vi "HighFrameRateRecording.vi"() -> ()   [LabVIEW 2014]
doc: "The LL Ring VI acquires images continuously and displays them in an image control using the low-level acquisition VIs. A ring initiates a continuous high-speed acquisition to multiple buffers and is appropriate for high-speed applications that perform processing on every image. Multiple buffers are useful when processing times vary depending on other applications and processing results .\n\nIMAQ Init initializes the device. IMAQ Configure List configures the buffer list with multiple buffers. IMAQ Create creates the image buffers. Call IMAQ Configure Buffer once for each buffer in the buffer list. IMAQ Start starts the acquisition, and IMAQ Extract Buffer ensures that the current image is not overwritten. An image control displays the image on the front panel. After exiting the loop, IMAQ Extract Buffer releases the last extracted buffer. IMAQ Close releases resources associated with the acquisition, and IMAQ Dispose frees the image buffer."
uses:
  <vilib>/vision/Avi.llb/IMAQ AVI2 Refnum.ctl
  <vilib>/vision/Avi.llb/IMAQ AVI2 Codec Path.ctl
  SubVI/Global_Video_Frame_Number.vi
panel:
  in  "Frames per file":i32
  out "AVI Refnum":T1
  out "Video recording":bool
  in  "Record? (Home bt.)":bool
  in  "codec index":i32=5
  out "Error (%)":dbl format="%#.4g"
  out "Missing Frames":i32
  out "Frame Number":u32=17170882
  out "codec":string="Y800 Uncompressed Grey Scale (NI Vision)"
  in  "AVI File Path":path=path "E:/Video/test/30fps.avi"
  out "Processed Frames/s":dbl=30.00968054211036 format="%#.1g"
  in  "Stop":bool
  out "Saved Frames":i32
  out "Image":T2(plugin-control)
  in  "camera selection":string="img0"
  in  "Buffer size (frames)":u32=1000
  # "ToDo:\n - add JSON output\n - andd indicator of _s# number"
  # "1.  Initialisation"
  # "Codec should be:\n\"Y800 Uncompressed Grey Scale\""
  # "Naming convention:\n - use the name above and add _s#.avi for videos\n - specs for saved videos is specified in name.json"
  # "2.  Recording"
  # "y"
  # "Record"
  # "x"
  # "Just Observe"
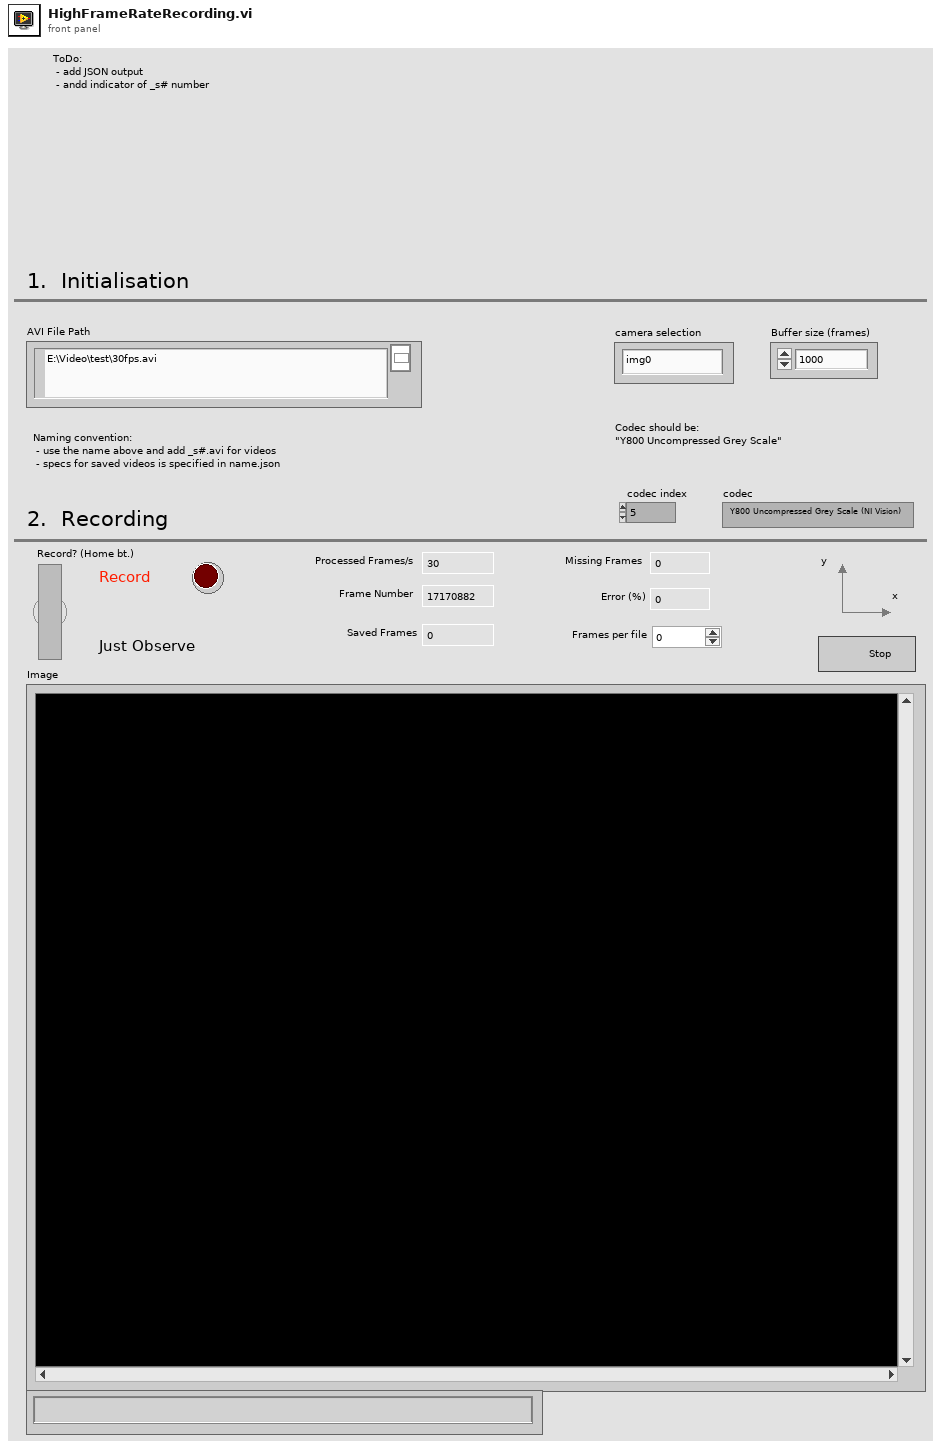
[diagram p1: front panel]
types:
  T1 = typedef "IMAQ AVI2 Refnum.ctl" = refnum<k20>
  T2 = typedef "IMAQ Image.ctl" = refnum<image>
  T3 = typedef "IMAQ AVI2 Codec Path.ctl" = u32
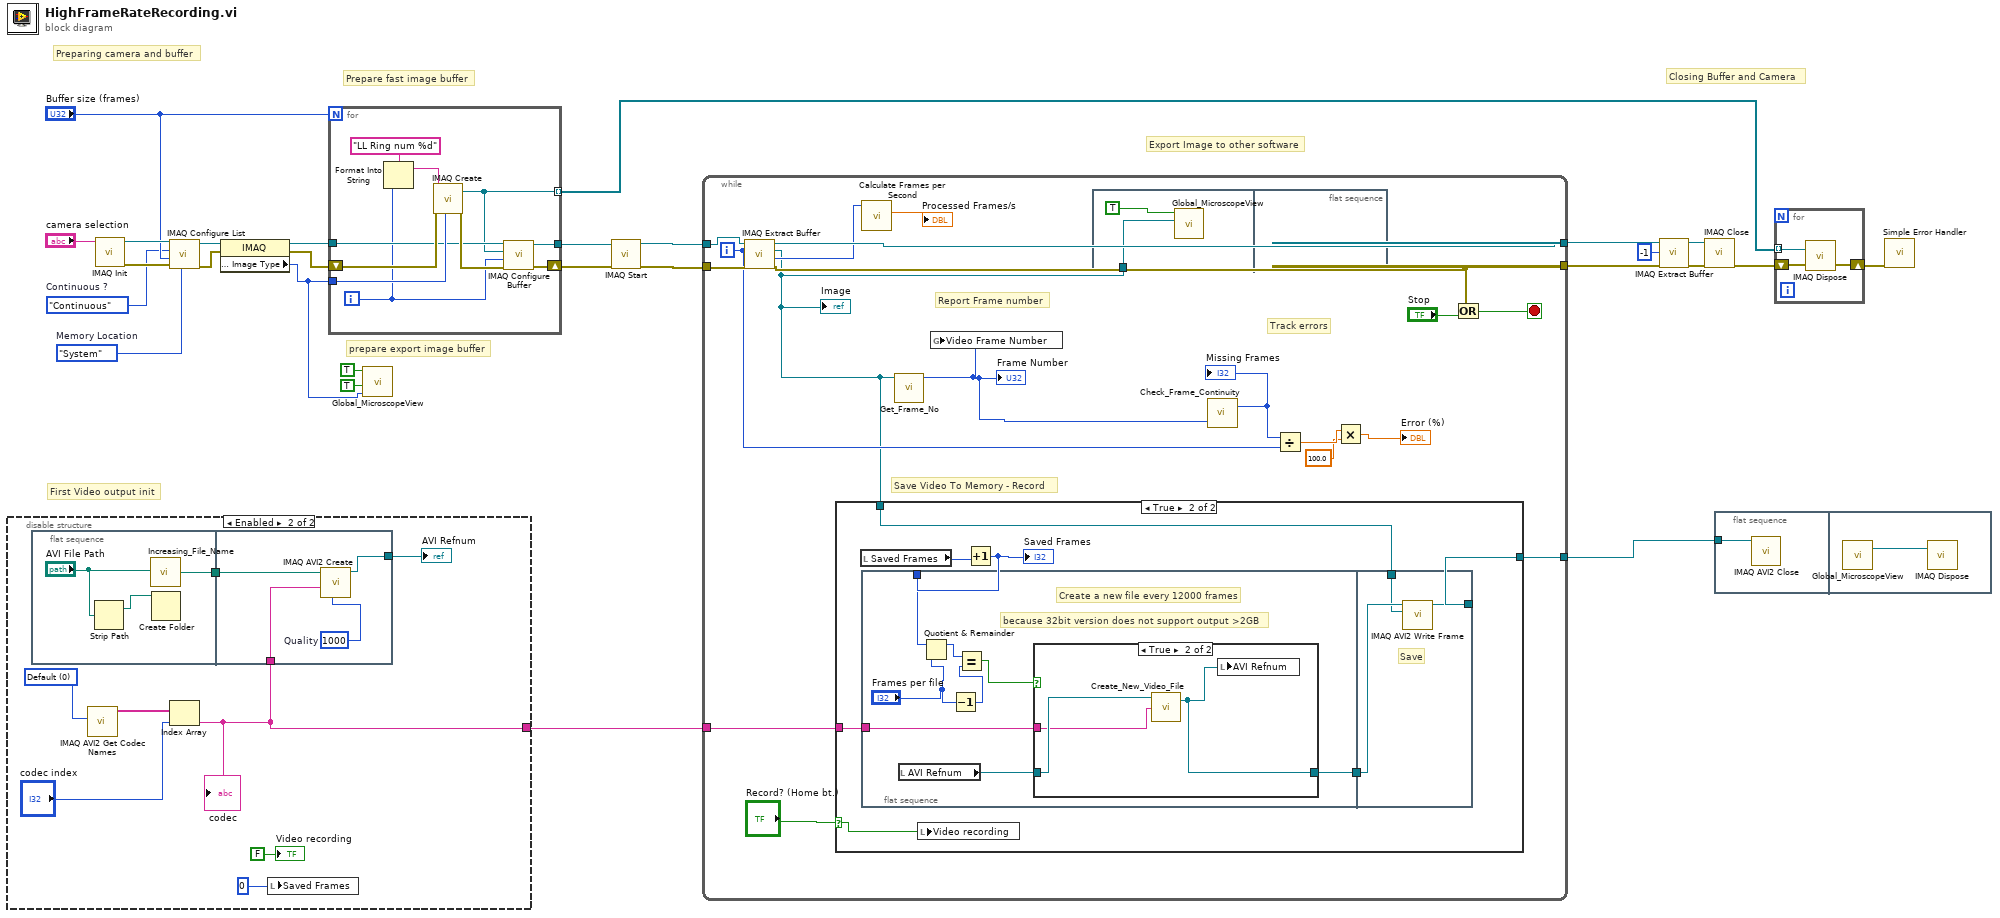
[diagram p0: block diagram]
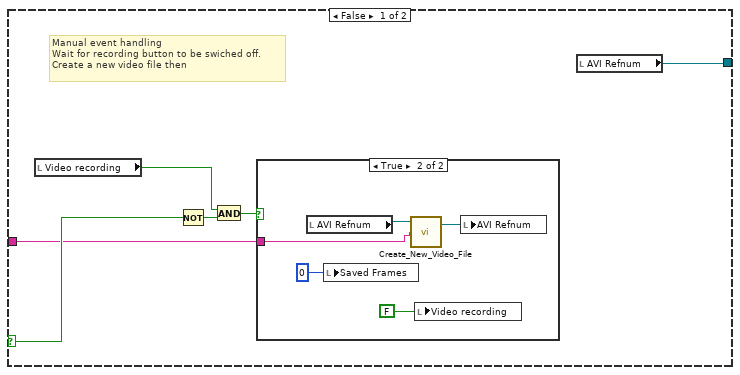
[diagram p3: hidden frame]
diagram:
  w9 = enum16{"System", "Onboard"}."System"  # Memory Location
  w8 = enum16{"One-Shot", "Continuous"}."Continuous"  # Continuous ?
  # "Export Image to other software"
  # "prepare export image buffer"
  # "Prepare fast image buffer"
  # "First Video output init"
  # "Closing Buffer and Camera"
  # "Preparing camera and buffer"
  n1 = disable-structure shown="Enabled" {
    disable-tunnel: [_ w28] -> w4
    frame Disabled {
    }
    frame Enabled {
      w35 = T3 0 items=["Default", "System", "Built in Vision"] ("Codec Source")
      n2 = flat-sequence {
        tunnel: [w38] -> w30
        tunnel: w30 -> [w40]
        tunnel: [w41] -> w29
        tunnel: w28 -> [w39]
        frame #0 {
          n3 = Strip Path(path="AVI File Path") -> (stripped path=w37:path)  [unwired: 1 out]
          n4 = call "Increasing_File_Name.vi"("Base AVI  path"="AVI File Path") -> ("Final AVI path"=w38:path)
          n5 = Create Folder(path (use dialog)=w37) -> ()  [unwired: 2 in, 3 out]
        }
        frame #1 {
          w42 = 1000  # Quality
          n6 = call "IMAQ AVI2 Create"("Quality"=w42, "Codec"=w39, "AVI Path"=w40) -> ("AVI Refnum"=w41:T1)  [unwired: 7 in, 1 out]
        }
      }
      n7 = call "IMAQ AVI2 Get Codec Names"("Codec Source"=w35) -> ("Codec Names"=w34:string[])  [unwired: 9 in, 1 out]
      n8 = Index Array(array=w34, index="codec index") -> (element=w28:string)
      "codec" <- w28
      n9 = local write "Saved Frames"(0 ("Saved Frames")) -> ()
      "AVI Refnum" <- w29
      "Video recording" <- FALSE ("Video recording")
    }
  }
  n10 = call <vilib>:"IMAQ Init.vi"("Interface Name"="camera selection") -> ("error out"=w26:errorcluster, "IMAQ Session Out"=w27:refnum<k11>)  [unwired: 1 in, 8 out]
  n11 = call <vilib>:"IMAQ Configure List.vi"("Memory Location"=w9, "error in (no error)"=w26, "Number of buffers"="Buffer size (frames)", "Continuous?"=w8, "IMAQ Session In"=w27) -> ("error out"=w22:errorcluster, "IMAQ Session Out"=w21:refnum<k11>)  [unwired: 1 in, 4 out]
  n12 = property class="IMAQ"(reference=w21, error in=w22) -> (reference out=w14:refnum<k11>, error out=w13:errorcluster, "Image Parameters : Image Type"=w1:u32)
  n13 = for {
    N: "Buffer size (frames)" -> [_]
    tunnel: [w52] -> w11
    tunnel: w1 -> [w50]
    tunnel: w14 -> [w47]
    shift-right: [w51] -> w10
    shift-left: w13 -> [w49]
    tunnel: [w43] -> w7 mode=indexing
    i -> [w44]
    n14 = Format Into String(format string="LL Ring num %d", w44) -> (resulting string=w46:string)  [unwired: 2 in, 1 out]
    n15 = call "IMAQ Create"("Image Name"=w46, "Image Type"=w50, "error in (no error)"=w49) -> ("New Image"=w43:T2, "error out"=w48:errorcluster)  [unwired: 1 in, 1 out]
    n16 = call <vilib>:"IMAQ Configure Buffer.vi"("error in (no error)"=w48, "Buffer Number"=w44, "Image In"=w43, "IMAQ Session In"=w47) -> ("error out"=w51:errorcluster, "IMAQ Session Out"=w52:refnum<k11>)  [unwired: 2 in, 4 out]
  }
  n17 = call "Global_MicroscopeView.vi"("Image Type"=w1, "Initialise"=TRUE, "Update Image"=TRUE) -> ()  [unwired: 1 in, 2 out]
  n18 = call <vilib>:"IMAQ Start.vi"("error in (no error)"=w10, "IMAQ Session In"=w11) -> ("error out"=w6:errorcluster, "IMAQ Session Out"=w17:refnum<k11>)  [unwired: 8 out]
  n19 = while {
    tunnel: [w68] -> w19
    tunnel: w17 -> [w69]
    tunnel: [w57] -> w18
    tunnel: w6 -> [w64]
    tunnel: [w56] -> w5
    tunnel: w4 -> [w55]
    i -> [w59]
    stop <- w70 stop-if-true
    # "Track errors"
    # "Report Frame number"
    # "Save Video To Memory - Record"
    n20 = call <vilib>:"IMAQ Extract Buffer.vi"("error in (no error)"=w64, "Buffer to extract"=w59, "IMAQ Session In"=w69) -> ("error out"=w57:errorcluster, "Buffer Number"=w65:i32, "Image Out"=w53:T2, "IMAQ Session Out"=w68:refnum<k11>)  [unwired: 5 out]
    "Image" <- w53
    n21 = case shown="True" "Record? (Home bt.)" {
      selector: "Record? (Home bt.)" -> [w75 w85]
      tunnel: [w78 w88] -> w56
      tunnel: w53 -> [_ w86]
      tunnel: w55 -> [w73 w84]
      frame False {
        # "Manual event handling\nWait for recording button to be swiched off.\nCreate a new video file then"
        n22 = local read "Video recording"() -> (w74:bool)
        n23 = Not(x=w75) -> (.not. x?=w76:bool)
        n24 = And(x=w74, y=w76) -> (x .and. y?=w77:bool)
        n25 = case shown="True" w77 {
          tunnel: w73 -> [_ w79]
          frame False {
          }
          frame True {
            n26 = local read "AVI Refnum"() -> (w82:T1)
            n27 = local write "Saved Frames"(0 ("Saved Frames")) -> ()
            n28 = call "Create_New_Video_File.vi"("Codec"=w79, "AVI Refnum IN"=w82) -> ("AVI Refnum OUT"=w83:T1)  [unwired: 1 in, 1 out]
            n29 = local write "Video recording"(FALSE ("Video recording")) -> ()
            n30 = local write "AVI Refnum"(w83) -> ()
          }
        }
        n31 = local read "AVI Refnum"() -> (w78:T1)
      }
      frame True {
        n32 = local read "Saved Frames"() -> (w90:i32)
        n33 = flat-sequence {
          tunnel: w89 -> [w96]
          tunnel: [w93] -> w87
          tunnel: w84 -> [w92]
          tunnel: [w105] -> w88
          tunnel: w87 -> [w104]
          tunnel: w86 -> [w103]
          frame #0 {
            # "because 32bit version does not support output >2GB"
            # "Create a new file every 12000 frames"
            n34 = local read "AVI Refnum"() -> (w94:T1)
            n35 = Quotient & Remainder(x=w96, y="Frames per file") -> (x-y*floor(x/y)=w98:i32)  [unwired: 1 out]
            n36 = Decrement(x="Frames per file") -> (x-1=w97:i32)
            n37 = Equal?(x=w98, y=w97) -> (x = y?=w95:bool)
            n38 = case shown="True" w95 {
              tunnel: w94 -> [w99 w102]
              tunnel: [w99 w101] -> w93
              tunnel: w92 -> [_ w100]
              frame False {
              }
              frame True {
                n39 = call "Create_New_Video_File.vi"("Codec"=w100, "AVI Refnum IN"=w102) -> ("AVI Refnum OUT"=w101:T1)  [unwired: 1 in, 1 out]
                n40 = local write "AVI Refnum"(w101) -> ()
              }
            }
          }
          frame #1 {
            # "Save"
            n41 = call "IMAQ AVI2 Write Frame"("Image"=w103, "AVI Refnum"=w104) -> ("AVI Refnum (duplicate)"=w105:T1)  [unwired: 7 in, 2 out]
          }
        }
        n42 = local write "Video recording"(w85) -> ()
        n43 = Increment(x=w90) -> (x+1=w89:i32)
        "Saved Frames" <- w89
      }
    }
    n44 = call <vilib>:"Calculate Frames per Second.vi"("Buffer Number"=w65) -> ("Processed Frames/s"=→"Processed Frames/s":dbl)  [unwired: 8 in, 2 out]
    n45 = call "Get_Frame_No.vi"("Image In"=w53) -> ("Frame Number"=w54:u32)  [unwired: 10 in]
    "Frame Number" <- w54
    n46 = global write "Global_Video_Frame_Number.vi" "Video Frame Number"(w54) -> ()
    n47 = flat-sequence {
      tunnel: w53 -> [w71]
      frame #0 {
        n48 = call "Global_MicroscopeView.vi"("New Image"=w71, "Update Image"=TRUE) -> ()  [unwired: 2 in, 2 out]
      }
      frame #1 {
      }
    }
    n49 = call "Check_Frame_Continuity.vi"("N"=w54) -> ("No of missed frames"=w60:i32)  [unwired: 1 in, 1 out]
    "Missing Frames" <- w60
    n50 = Divide(x=w60, y=w59) -> (x/y=w62:dbl)
    n51 = Multiply(x=w62, y=100.0) -> (x*y=→"Error (%)":dbl)
    n52 = Or(x=w57, y="Stop") -> (x .or. y?=w70:bool)
  }
  n53 = call <vilib>:"IMAQ Extract Buffer.vi"("error in (no error)"=w18, "Buffer to extract"=-1, "IMAQ Session In"=w19) -> ("error out"=w16:errorcluster, "IMAQ Session Out"=w15:refnum<k11>)  [unwired: 7 out]
  n54 = call <vilib>:"IMAQ Close.vi"("error in (no error)"=w16, "IMAQ Session In"=w15) -> ("error out"=w23:errorcluster)  [unwired: 9 out]
  n55 = flat-sequence {
    tunnel: w5 -> [w106]
    frame #0 {
      n56 = call "IMAQ AVI2 Close"("AVI Refnum"=w106) -> ()  [unwired: 10 in, 1 out]
    }
    frame #1 {
      n57 = call "Global_MicroscopeView.vi"() -> ("MicroscopeView"=w107:T2)  [unwired: 4 in, 1 out]
      n58 = call "IMAQ Dispose"("Image"=w107) -> ()  [unwired: 2 in, 4 out]
    }
  }
  n59 = for {
    tunnel: w7 -> [w110] mode=indexing
    shift-right: [w108] -> w24
    shift-left: w23 -> [w109]
    n60 = call "IMAQ Dispose"("Image"=w110, "error in (no error)"=w109) -> ("error out"=w108:errorcluster)  [unwired: 1 in, 3 out]
  }
  n61 = call <vilib>:"Simple Error Handler.vi"("error in (no error)"=w24) -> ()  [unwired: 1 in, 8 out]
